vi "Launch NIVS.vi"() -> (0 "error out":errorcluster)   [LabVIEW 2013, in "MiscHelperVIs.lvlib"]
uses:
  MiscHelperVIs.lvlib
  <vilib>/NI Veristand/Execution/Workspace/NI_VS Workspace ExecutionAPI.lvlib
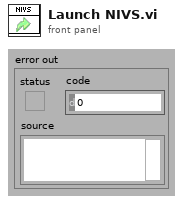
[diagram p1: front panel]
types:
  T1 = typedef "NI_VS Workspace ExecutionAPI.lvlib/WorkspaceAPI.ctl" = refnum<k24>
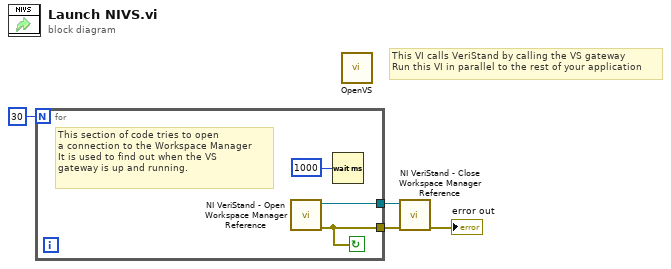
[diagram p0: block diagram]
diagram:
  # "This VI calls VeriStand by calling the VS gateway\nRun this VI in parallel to the rest of your application"
  n1 = for {
    N: 30 -> [_]
    tunnel: [w6] -> w3
    tunnel: [w5] -> w4
    stop <- w5 continue-if-true
    # "This section of code tries to open \na connection to the Workspace Manager\nIt is used to find out when the VS\ngateway is up and running."
    n2 = call <vilib>:"NI VeriStand - Open Workspace Manager Reference.vi"() -> ("error out"=w5:errorcluster, "WorkspaceManager"=w6:T1)  [unwired: 10 in]
    n3 = Wait (ms)(milliseconds to wait=u32 1000) -> ()  [unwired: 1 out]
  }
  n4 = call "OpenVS.vi"() -> ()  [unwired: 12 in]
  n5 = call <vilib>:"NI VeriStand - Close Workspace Manager Reference.vi"("error in (no error)"=w4, "WorkspaceManager"=w3) -> ("error out"=→"error out":errorcluster)  [unwired: 9 in]
